vi "CamSort Marble Sorter.vi"() -> ()   [LabVIEW 2024]
uses:
  39fd810c-f368-4577-b106-3b32b6a7f5d5.vi
  3e8d7108-7736-4374-987d-be3cc1b98066.vi
  e53b00cb-0bb5-45c7-b05d-b2842b2e883f.vi
  fdf2dff2-e640-4ee4-9198-689981333d90.vi
  <vilib>/DAQmx/create/channels.llb/DAQmx Create Channel (CO-Pulse Generation-Frequency).vi
panel:
  in  "stop":bool
  in  "counter 3":tag
  in  "counter 2":tag
  out "Classes (Color Classification 1)":string[](array[string])
  in  "counter":tag
  out "Number of Matches (Pattern Matching 1)":i32
  in  "Parameters (Pattern Matching 1)":T1={"Number of Matches Requested"=1, "Minimum Match Score"=800.0, "Angle Ranges"=[{"Start Angle"=-5.0, "End Angle"=5.0}]}
  in  "Stop (F)":bool
  out "Image Out":T2(plugin-control)
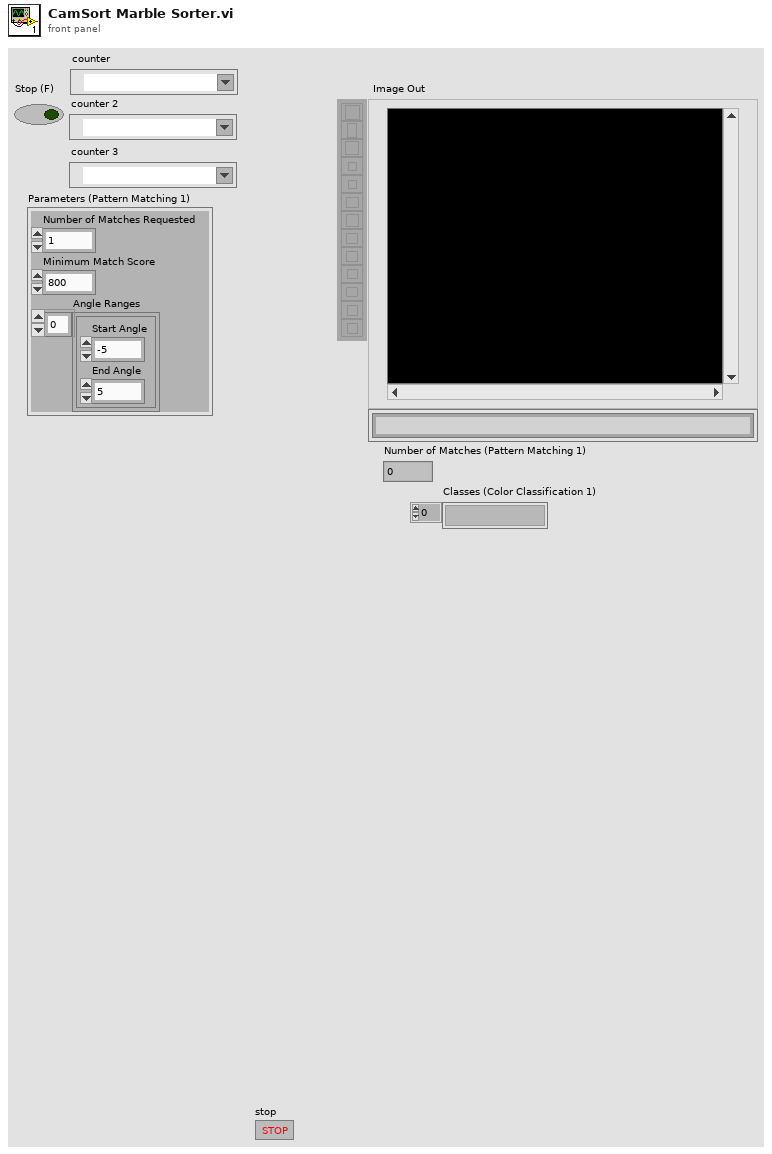
[diagram p1: front panel]
types:
  T1 = cluster{"Number of Matches Requested":i32, "Minimum Match Score":sgl, "Angle Ranges":cluster{"Start Angle":sgl, "End Angle":sgl}[]}
  T2 = typedef "IMAQ Image.ctl" = refnum<image>
  T3 = typedef "Image Type" = u32
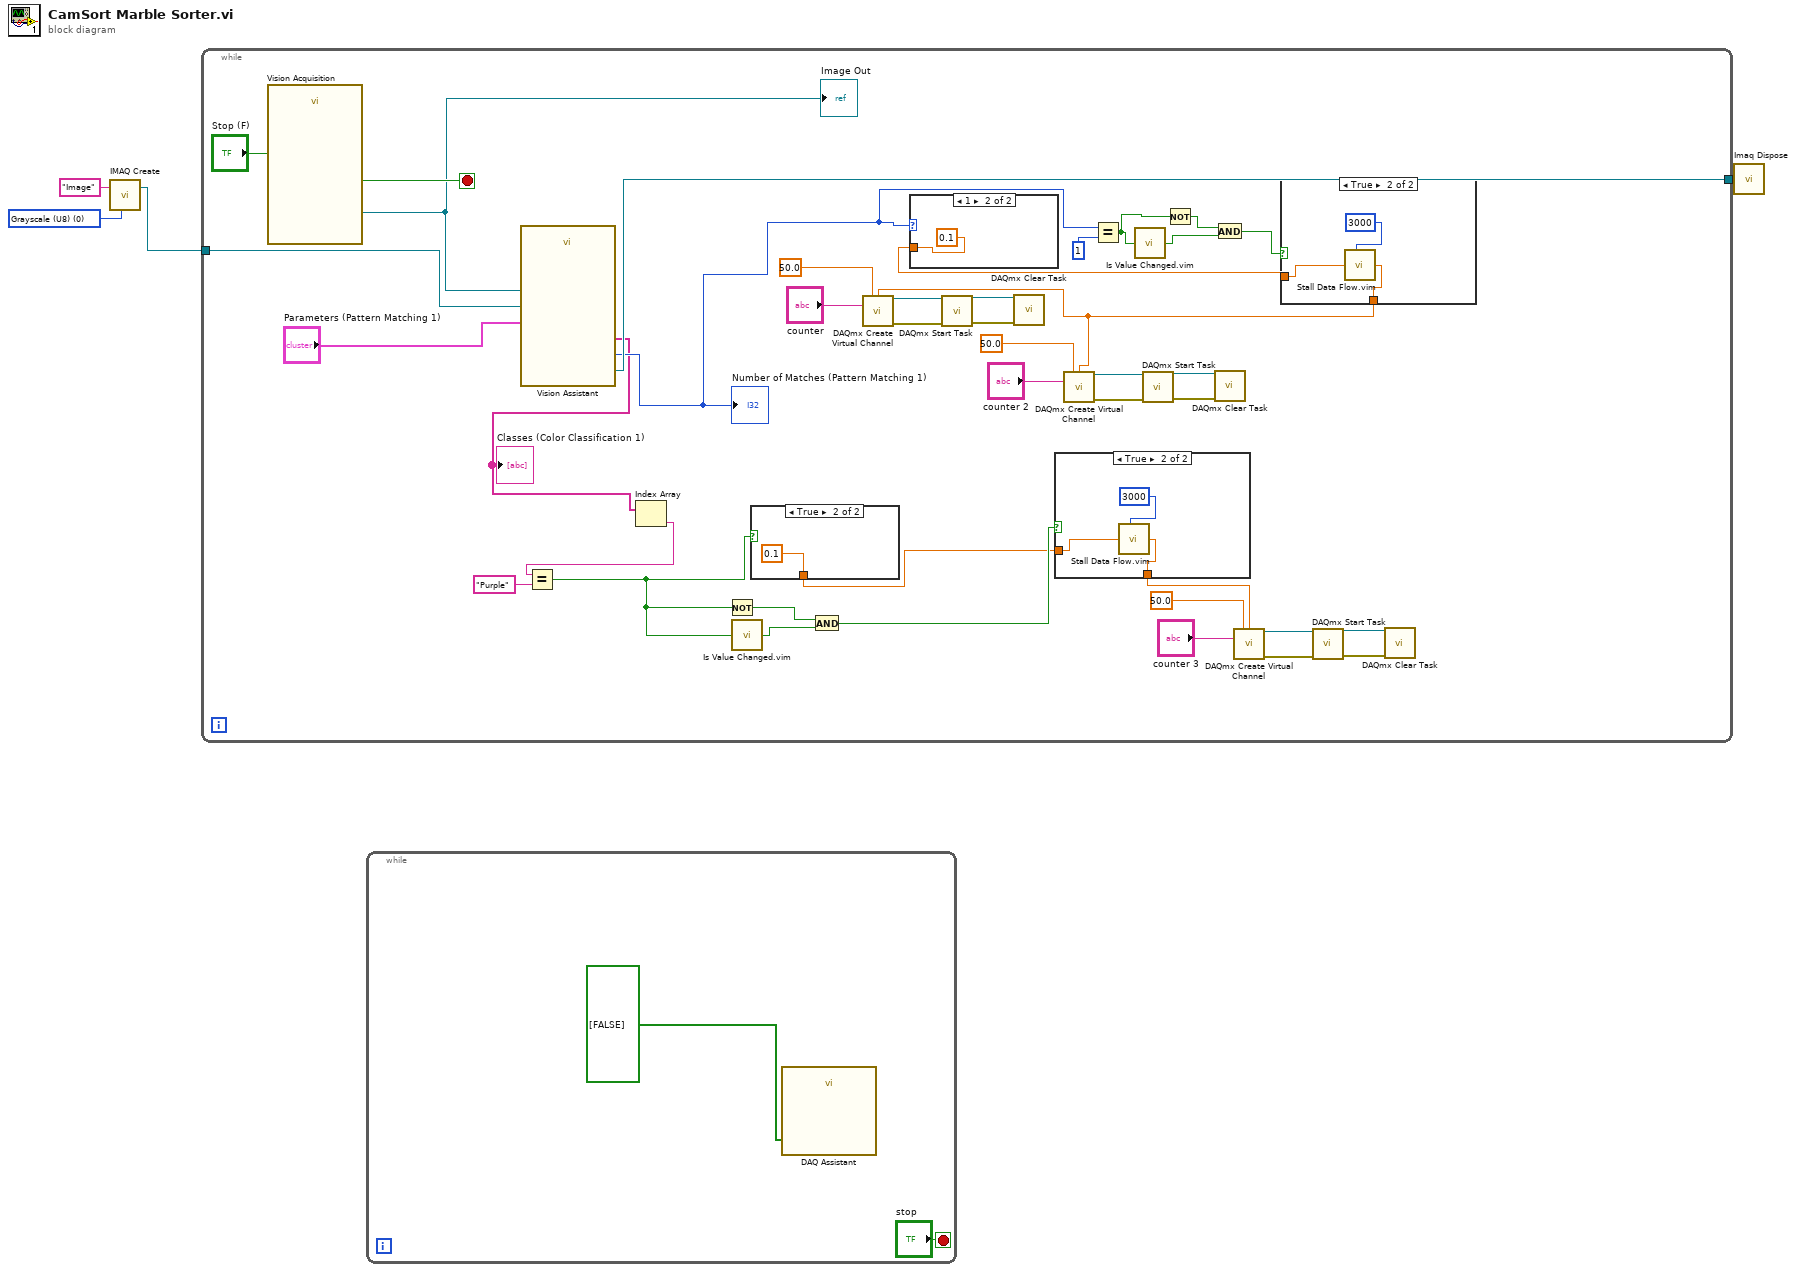
[diagram p0: block diagram]
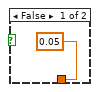
[diagram p3: hidden frame]
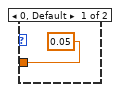
[diagram p5: hidden frame]
diagram:
  w4 = T3 0 items=["Grayscale (U8)", "Grayscale (I16)", "Grayscale (SGL)", "Complex (CSG)", "RGB (U32)", "HSL (U32)", "RGB (U64)", "Grayscale (U16)"] ("Image Type")
  n1 = call "IMAQ Create"("Image Name"="Image", "Image Type"=w4) -> ("New Image"=w2:T2)  [unwired: 3 in, 1 out]
  n2 = while {
    tunnel: w2 -> [w42]
    tunnel: [w40] -> w1
    stop <- w44 stop-if-true
    n3 = call "Vision Acquisition"("Stop (F)"="Stop (F)") -> ("Image Out"=w43:T2, "Stopped"=w44:bool)  [unwired: 24 in, 1 out]
    "Image Out" <- w43
    n4 = call "Vision Assistant"("Image In"=w43, "Image Dst"=w42, "Parameters (Pattern Matching 1)"="Parameters (Pattern Matching 1)") -> ("Image Out"=w40:T2, "Classes (Color Classification 1)"=w19:string[], "Number of Matches (Pattern Matching 1)"=w31:i32)  [unwired: 21 in, 1 out]
    "Number of Matches (Pattern Matching 1)" <- w31
    "Classes (Color Classification 1)" <- w19
    n5 = Index Array(array=w19) -> (element=w18:string)  [unwired: 1 in]
    n6 = Equal?(x=w18, y="Purple") -> (x = y?=w14:bool)
    n7 = Not(x=w14) -> (.not. x?=w16:bool)
    n8 = call "Is Value Changed.vim"("value"=w14) -> ("changed or first call?"=w15:bool)
    n9 = case shown="True" w14 {
      tunnel: [0.05 0.1] -> w12
      frame False {
      }
      frame True {
      }
    }
    n10 = And(x=w16, y=w15) -> (x .and. y?=w13:bool)
    n11 = case shown="1" w31 {
      tunnel: [0.05 0.1] -> w22
      frame 0, Default {
      }
      frame 1 {
      }
    }
    n12 = case shown="True" w13 {
      tunnel: w12 -> [w46 w48]
      tunnel: [w46 w47] -> w5
      frame False {
      }
      frame True {
        n13 = call "Stall Data Flow.vim"("value in"=w48, "milliseconds to wait"=3000) -> ("value out"=w47:dbl)  [unwired: 1 out]
      }
    }
    n14 = Equal?(x=w31, y=1) -> (x = y?=w29:bool)
    n15 = call "Is Value Changed.vim"("value"=w29) -> ("changed or first call?"=w32:bool)
    n16 = Not(x=w29) -> (.not. x?=w33:bool)
    n17 = And(x=w33, y=w32) -> (x .and. y?=w28:bool)
    n18 = call-poly <vilib>:"DAQmx Create Virtual Channel.vi"("frequency"=50.0 ("Frequency"), "duty cycle"=w5, "counter"="counter 3") -> ("task out"=w10:refnum<k21>, "error out"=w9:errorcluster)  [unwired: 11 in]
    n19 = case shown="True" w28 {
      tunnel: w22 -> [w52 w54]
      tunnel: [w52 w53] -> w20
      frame False {
      }
      frame True {
        n20 = call "Stall Data Flow.vim"("value in"=w54, "milliseconds to wait"=3000) -> ("value out"=w53:dbl)  [unwired: 1 out]
      }
    }
    n21 = call-poly <vilib>:"DAQmx Create Virtual Channel.vi"("frequency"=50.0 ("Frequency"), "duty cycle"=w20, "counter"="counter") -> ("task out"=w37:refnum<k21>, "error out"=w36:errorcluster)  [unwired: 11 in]
    n22 = call <vilib>:"DAQmx Start Task.vi"("task/channels in"=w37, "error in"=w36) -> ("task out"=w35:refnum<k21>, "error out"=w34:errorcluster)  [unwired: 12 in]
    n23 = call <vilib>:"DAQmx Clear Task.vi"("task in"=w35, "error in"=w34) -> ()  [unwired: 13 in, 1 out]
    n24 = call-poly <vilib>:"DAQmx Create Virtual Channel.vi"("frequency"=50.0 ("Frequency"), "duty cycle"=w20, "counter"="counter 2") -> ("task out"=w26:refnum<k21>, "error out"=w25:errorcluster)  [unwired: 11 in]
    n25 = call <vilib>:"DAQmx Start Task.vi"("task/channels in"=w26, "error in"=w25) -> ("task out"=w24:refnum<k21>, "error out"=w23:errorcluster)  [unwired: 12 in]
    n26 = call <vilib>:"DAQmx Clear Task.vi"("task in"=w24, "error in"=w23) -> ()  [unwired: 13 in, 1 out]
    n27 = call <vilib>:"DAQmx Start Task.vi"("task/channels in"=w10, "error in"=w9) -> ("task out"=w8:refnum<k21>, "error out"=w7:errorcluster)  [unwired: 12 in]
    n28 = call <vilib>:"DAQmx Clear Task.vi"("task in"=w8, "error in"=w7) -> ()  [unwired: 13 in, 1 out]
  }
  n29 = while {
    stop <- "stop" stop-if-true
    n30 = call "DAQ Assistant"("data"=bool[] [FALSE]) -> ()  [unwired: 17 in, 2 out]
  }
  n31 = call "Imaq Dispose"("Image"=w1) -> ()  [unwired: 5 in, 1 out]
